vi "ACTUATOR ENC SPI RW.vi"(2 "CPOL":bool, 3 "Data to Write":u8[](array[numeric])=[0, 0, 0, 0, 0, 0, 0, 0, 0, 0] format="%x", 4 "Frames to Write":u8, 5 "SPI Frequency (KHz)":u16) -> (0 "Data Read":u8[](array[numeric]) format="%x", 1 "Frames Read":u8)   [LabVIEW 2019]
uses:
  <vilib>/Platform/TimedLoop/XDataNode/timing_clust.ctl
  <vilib>/Platform/TimedLoop/XDataNode/nitl_modes.ctl
  <vilib>/Platform/TimedLoop/XDataNode/wakeup.ctl
  <vilib>/rvi/DataTransferAndStorage/Container/Common/niFpgaContainerExecOnDevCompGetState.vi
  <vilib>/rvi/Emulation/niFpgaEmulationIsFPGAContextNoSignature.vi
  <vilib>/rvi/Emulation/niFpgaSctlEmulationGetInTimedLoop.vi
  <vilib>/rvi/errors/niFpgaSetErrorForExecOnDevCompSimple.vi
  <vilib>/rvi/eio/common/nirviEmuReportErrorAndStop.vi
  <vilib>/rvi/DataTransferAndStorage/Container/Common/niFpgaContainerGetUniqueNameForEmu.vi
  <vilib>/rvi/FIFO/Fifo_Resource/nirvififoEmulationSetSize.vi
  <vilib>/rvi/FIFO/Fifo_Resource/nirviFifoEmulationQueueMgr.vi
  <instcachedir>/0/nirviFifoEmulationQueueMgr_E5CAEC123FF24DC58D834DCA3CDAA9B5.lvgen/nirviFifoEmulationQueueMgr_E5CAEC123FF24DC58D834DCA3CDAA9B5_001.vi
  <vilib>/rvi/FIFO/Fifo_Resource/nirvififoEmulationDetermineInputValidOut.vi
  <vilib>/rvi/FIFO/Fifo_Resource/nirvififoEmulationCreateLock.vi
  <vilib>/rvi/Emulation/niFpgaProcessEmulError.vi
  <vilib>/rvi/FIFO/Fifo_Resource/nirvififoEmulationObtainLock.vi
  <vilib>/rvi/FIFO/Fifo_Resource/nirvififoEmulationReleaseLock.vi
  <vilib>/rvi/occurrence/nirviWaitOnOccurrenceBase.vi
  <vilib>/rvi/errors/nirviReportUnexpectedCaseInternalError.vi
  <vilib>/rvi/errors/nirviReportUnexpectedCaseInternalError (U32).vi
  <vilib>/Utility/error.llb/Clear Errors.vi
  <vilib>/rvi/interface/RandomDataEmulation/niFpgaRandomDataHandleErrors.vi
  <vilib>/rvi/Emulation/niFpgaEmulationReportErrorSimple.vi
  <vilib>/rvi/Emulation/niFpgaGetClockAttributes.vi
  <vilib>/rvi/Emulation/niFpgaCriticalErrorInLSC.vi
  <vilib>/rvi/eio/common/nirviEmuTemplateMethod_errors.vi
  <vilib>/rvi/DataTransferAndStorage/Container/XNode/niFpgaContainer.xnode
  <vilib>/rvi/FIFO/Fifo_Resource/niFpgaFifoEmulationRefIn.vi
  <vilib>/platform/TimedLoop/XDataNode/XDataNode.xnode
  <vilib>/rvi/FXPMathLib/basic elements/FxpDiscreteDelay/XNode/nifxpmath_DiscreteDelay.xnode
  <vilib>/eio/EIONode/EIONode.xnode
  <vilib>/Platform/TimedLoop/XDataNode/XDNodeRunTimeDep.lvlib
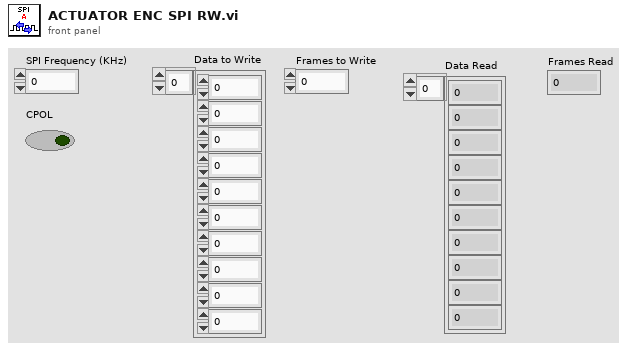
[diagram p1: front panel]
types:
  T1 = cluster{"SCLK":refnum<k21>, "MISO":refnum<k21>, "MOSI":refnum<k21>, "TxBuffer":refnum<k21>, "RxBuffer":refnum<k21>}
  T2 = typedef "XDNodeRunTimeDep.lvlib/timing_clust.ctl" = cluster{"Expected End [f-1]":u64, "Actual End [f-1]":u64, "Finished Late? [f-1]":bool, "Expected End [i-1]":u64, "Actual End [i-1]":u64, "Finished Late? [i-1]":bool, "Expected Start [i]":u64, "Actual Start [i]":u64, "Expected Start [f]":u64, "Actual Start [f]":u64, "Source Name":string, "Structure Name":string, "Period":i64, "Deadline":i64, "Offset":i64, "Start":i64, "Priority":i32, "Timeout":i32, "Mode":T3, "Wakeup Reason":T4, "Error":errorcluster, "Source Type":string, "Secondary Source Type":string, "Global End Time":u64, "Global Start Time":u64, "Frame Duration":u64, "Iteration Duration":u64, "Assigned CPU":i32, "I/O Scan Engine Mode":u32}
  T3 = typedef "XDNodeRunTimeDep.lvlib/nitl_modes.ctl" = enum32{"No Change", "Process missed periods, maintain original phase", "Discard missed periods, maintain original phase", "Process missed periods, ignore original phase", "Discard missed periods, ignore original phase"}
  T4 = typedef "XDNodeRunTimeDep.lvlib/wakeup.ctl" = enum32{"Normal", "Aborted", "Asynchronous wakeup", "Timing source error", "Timed loop error", "Timeout"}
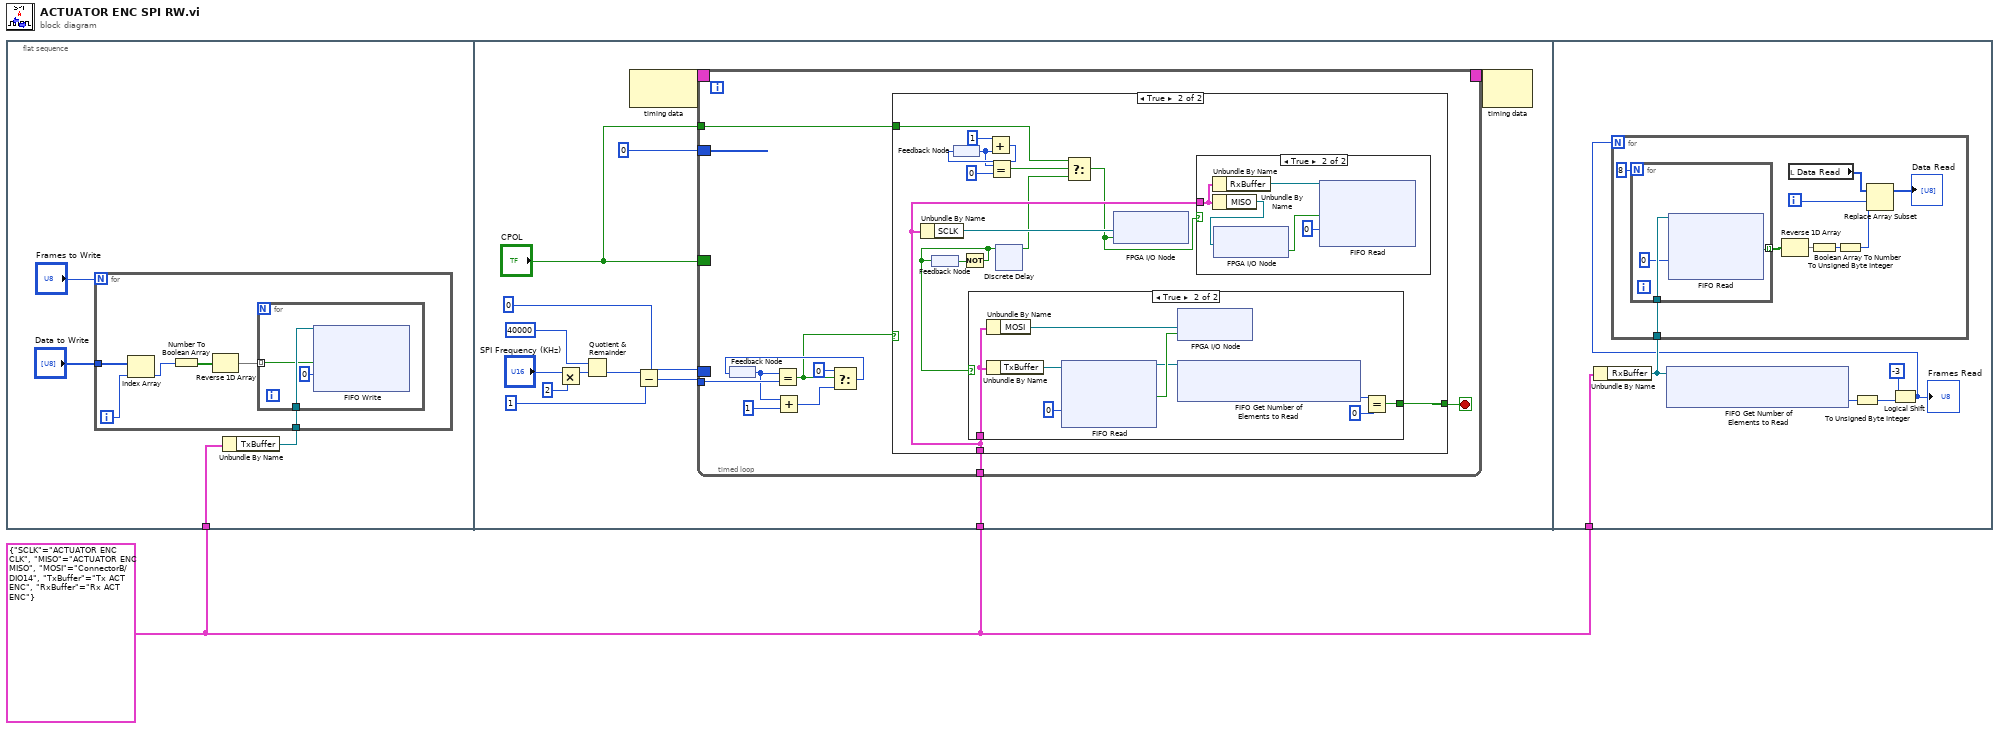
[diagram p0: block diagram]
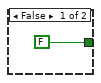
[diagram p2: hidden frame]
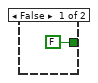
[diagram p4: hidden frame]
diagram:
  w1 = T1 {"SCLK"="ACTUATOR ENC CLK", "MISO"="ACTUATOR ENC MISO", "MOSI"="ConnectorB/DIO14", "TxBuffer"="Tx ACT ENC", "RxBuffer"="Rx ACT ENC"}
  n1 = flat-sequence {
    tunnel: w1 -> [w4]
    tunnel: w1 -> [w20]
    tunnel: w1 -> [w76]
    frame #0 {
      n2 = Unbundle By Name(w4) -> ("TxBuffer"=w3:refnum<k21>)
      n3 = for {
        N: "Frames to Write" -> [_]
        tunnel: "Data to Write" -> [w10]
        tunnel: w3 -> [w11]
        i -> [w9]
        n4 = Index Array(array=w10, index=w9) -> (element=w8:u8)
        n5 = Number To Boolean Array(number=w8) -> (Boolean array=w7:bool[])
        n6 = Reverse 1D Array(array=w7) -> (reversed array=w6:bool[])
        n7 = for {
          tunnel: w11 -> [w14]
          tunnel: w6 -> [w13] mode=indexing
          n8 = xnode ("FIFO Write")("Element"=w13, "Timeout"=0, "FIFO In"=w14) -> ()  [unwired: 2 out]
        }
      }
    }
    frame #1 {
      n9 = Multiply(x="SPI Frequency (KHz)", y=u16 2) -> (x*y=w18:u16)
      n10 = Quotient & Remainder(x=u16 40000, y=w18) -> (floor(x/y)=w23:u16)  [unwired: 1 out]
      n11 = node-c288() -> (w27:T2)  [unwired: 1 in]
      n12 = Subtract(x=w23, y=u16 1) -> (x-y=w21:u16)
      n13 = timed-loop {
        timing: w27 -> [_]
        timing-out: [_] -> w26
        tunnel: w21 -> [w37]
        border: u16 0 -> [_]
        tunnel: w20 -> [w30]
        border: "CPOL" -> [_]
        border: u16 0 -> [_]
        tunnel: "CPOL" -> [w28]
        stop <- w29 stop-if-true
        n14 = feedback #1() -> (w34:u16)
        n15 = Equal?(x=w34, y=w37) -> (x = y?=w31:bool)
        n16 = Add(x=w34, y=u16 1) -> (x+y=w32:u16)
        n17 = Select(t=u16 0, s=w31, f=w32) -> (s? t:f=w35:u16)
        n18 = feedback-in #1(w35) -> ()
        n19 = case shown="True" w31 {
          tunnel: w30 -> [_ w49]
          tunnel: [FALSE w50] -> w29
          tunnel: w28 -> [_ w39]
          frame False {
          }
          frame True {
            n20 = Unbundle By Name(w49) -> ("SCLK"=w51:refnum<k21>)
            n21 = feedback #2() -> (w48:bool)
            n22 = feedback #3() -> (w43:u16)
            n23 = Not(x=w48) -> (.not. x?=w47:bool)
            n24 = feedback-in #2(w47) -> ()
            n25 = case shown="True" w47 {
              tunnel: w49 -> [_ w62]
              tunnel: [FALSE w58] -> w50
              frame False {
              }
              frame True {
                n26 = Unbundle By Name(w62) -> ("MOSI"=w64:refnum<k21>)
                n27 = Unbundle By Name(w62) -> ("TxBuffer"=w66:refnum<k21>)
                n28 = xnode ("FIFO Read")("Timeout"=0, "FIFO In"=w66) -> ("Element"=w63:bool, "FIFO Out"=w61:refnum<k21>)  [unwired: 1 out]
                n29 = xnode "FPGA I/O Node"("I/O Item"=w63, "FPGA I/O In"=w64) -> ()  [unwired: 1 out]
                n30 = xnode ("FIFO Get Number of Elements to Read")("FIFO In"=w61) -> ("Number of Elements to Read"=w60:u32)  [unwired: 1 out]
                n31 = Equal?(x=w60, y=u32 0) -> (x = y?=w58:bool)
              }
            }
            n32 = Add(x=u16 1, y=w43) -> (x+y=w45:u16)
            n33 = feedback-in #3(w45) -> ()
            n34 = Equal?(x=w43, y=u16 0) -> (x = y?=w42:bool)
            n35 = xnode ("Discrete Delay")("D"=w47) -> ("Q"=w40:bool)
            n36 = Select(t=w39, s=w42, f=w40) -> (s? t:f=w41:bool)
            n37 = xnode "FPGA I/O Node"("I/O Item"=w41, "FPGA I/O In"=w51) -> ()  [unwired: 1 out]
            n38 = case shown="True" w41 {
              tunnel: w49 -> [_ w55]
              frame False {
              }
              frame True {
                n39 = Unbundle By Name(w55) -> ("RxBuffer"=w54:refnum<k21>)
                n40 = Unbundle By Name(w55) -> ("MISO"=w56:refnum<k21>)
                n41 = xnode "FPGA I/O Node"("FPGA I/O In"=w56) -> ("I/O Item"=w53:bool)  [unwired: 1 out]
                n42 = xnode ("FIFO Read")("Element"=w53, "Timeout"=0, "FIFO In"=w54) -> ()  [unwired: 2 out]
              }
            }
          }
        }
      }
      n43 = node-c288(w26) -> ()  [unwired: 1 out]
    }
    frame #2 {
      n44 = Unbundle By Name(w76) -> ("RxBuffer"=w75:refnum<k21>)
      n45 = xnode ("FIFO Get Number of Elements to Read")("FIFO In"=w75) -> ("Number of Elements to Read"=w74:u32)  [unwired: 1 out]
      n46 = To Unsigned Byte Integer(number=w74) -> (unsigned 8bit integer=w71:u8)
      n47 = Logical Shift(y=i16 -3, x=w71) -> (x << y=w72:u8)
      "Frames Read" <- w72
      n48 = for {
        N: w72 -> [_]
        tunnel: w75 -> [w85]
        i -> [w81]
        n49 = for {
          N: 8 -> [_]
          tunnel: w85 -> [w88]
          tunnel: [w86] -> w83 mode=indexing
          n50 = xnode ("FIFO Read")("Timeout"=0, "FIFO In"=w88) -> ("Element"=w86:bool)  [unwired: 2 out]
        }
        n51 = Reverse 1D Array(array=w83) -> (reversed array=w77:bool[])
        n52 = local read "Data Read"() -> (w82:u8[])
        n53 = Boolean Array To Number(Boolean array=w77) -> (number=w80:u8)
        n54 = To Unsigned Byte Integer(number=w80) -> (unsigned 8bit integer=w79:u8)
        n55 = Replace Array Subset(array=w82, new element=w79, index=w81) -> (→"Data Read":u8[])
      }
    }
  }
